vi "getEnumValues.vi"(0 "Enum reference":refnum<vi>, 1 "error in (no error)":errorcluster) -> (2 "Enum labels":string[](array[string]), 3 "Enum values":u16[](array[numeric]), 4 "error out":errorcluster)   [LabVIEW 2015]
doc: "Get the labels and values of a generic enum control"
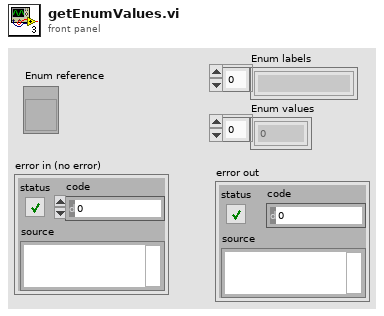
[diagram p1: front panel]
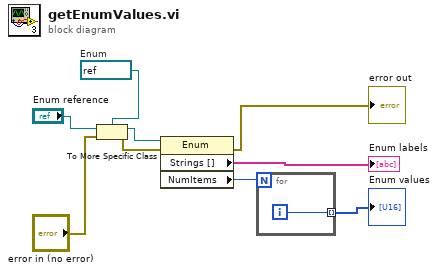
[diagram p0: block diagram]
diagram:
  w8 = refnum<vi> refnum  # Enum
  n1 = To More Specific Class(target class=w8, reference="Enum reference", error in="error in (no error)") -> (specific class reference=w7:refnum<vi>, error out=w6:errorcluster)
  n2 = property class="Enum"(reference=w7, error in=w6) -> (error out=→"error out":errorcluster, "Strings []"=→"Enum labels":string[], "NumItems"=w3:u32)  [unwired: 1 out]
  n3 = for {
    N: w3 -> [_]
    tunnel: [w10] -> w2 mode=indexing
    i -> [w10]
  }
  "Enum values" <- w2
